vi "Shutter Experiments.vi"(8 "Laser Shutter":enum32{"GFP", "Cy3 Long Pass", "Cy3", "Cy5"}(radio)) -> ()   [LabVIEW 2014]
uses:
  global current shutter.vi
panel:
  out "Current Wheel Position":string
  in  "Wheel Speed":u8=1 min=1 max=7 step=1
  in  "stop":bool
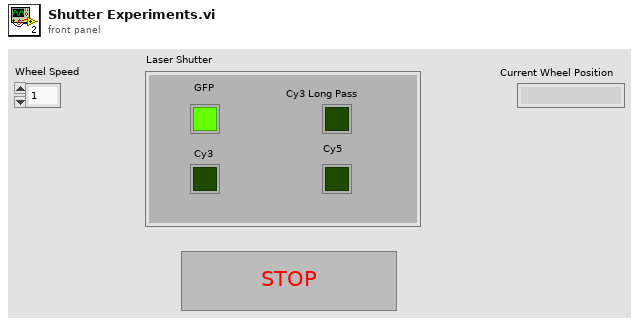
[diagram p1: front panel]
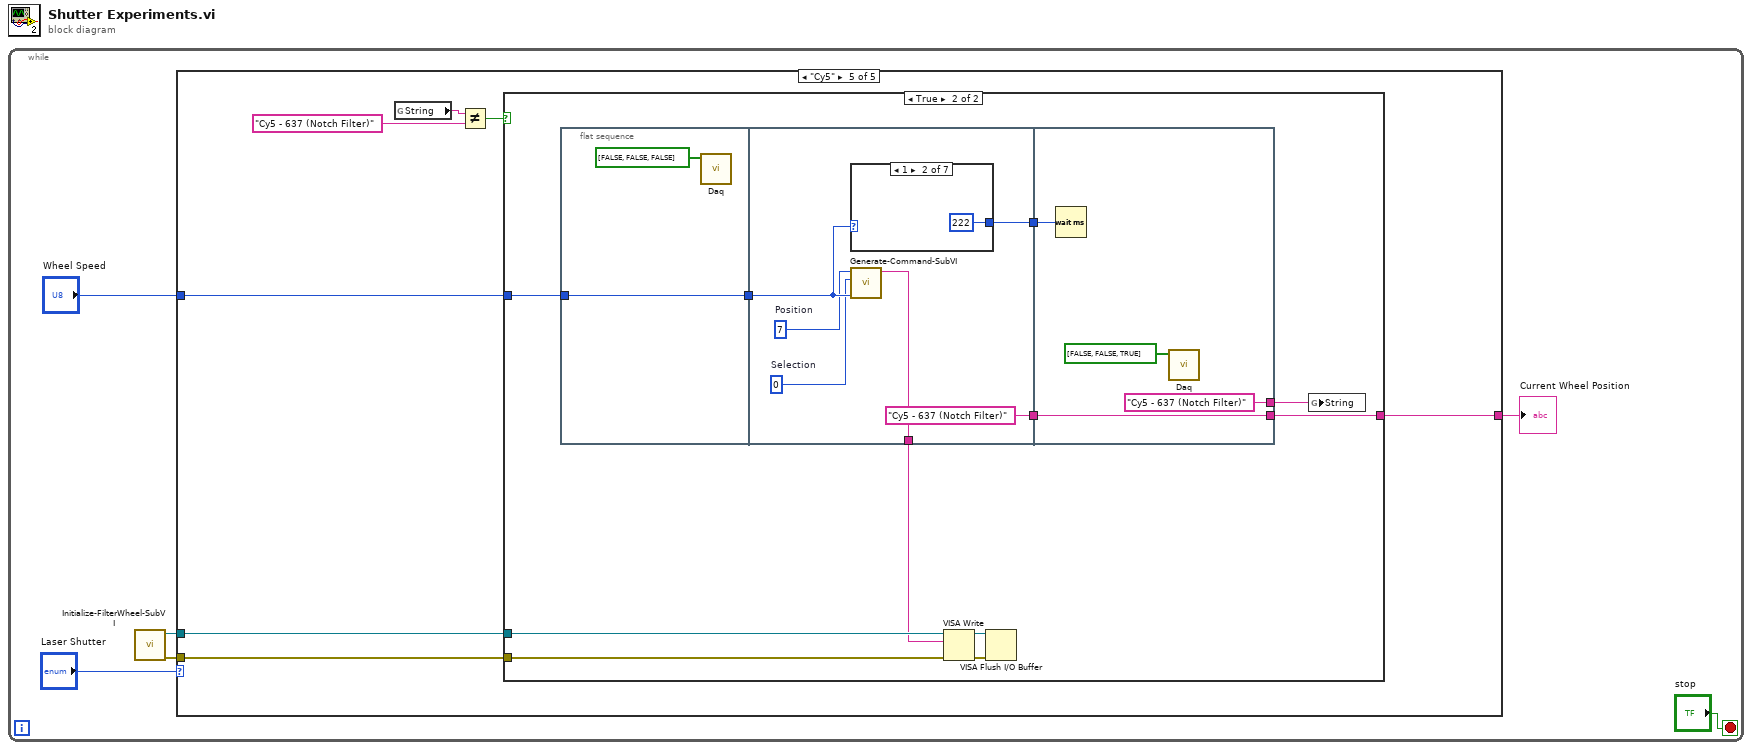
[diagram p0: block diagram]
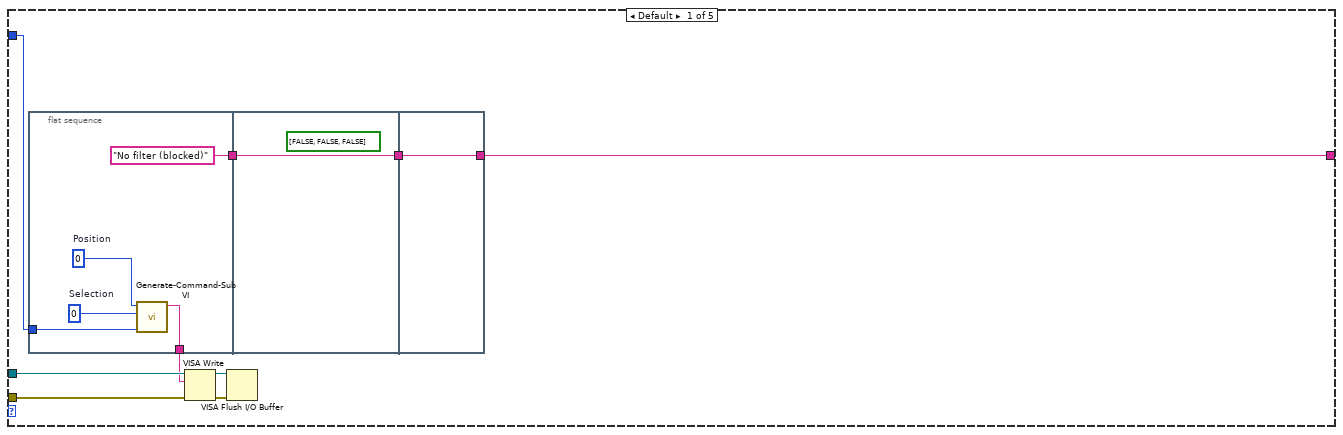
[diagram p2: hidden frame]
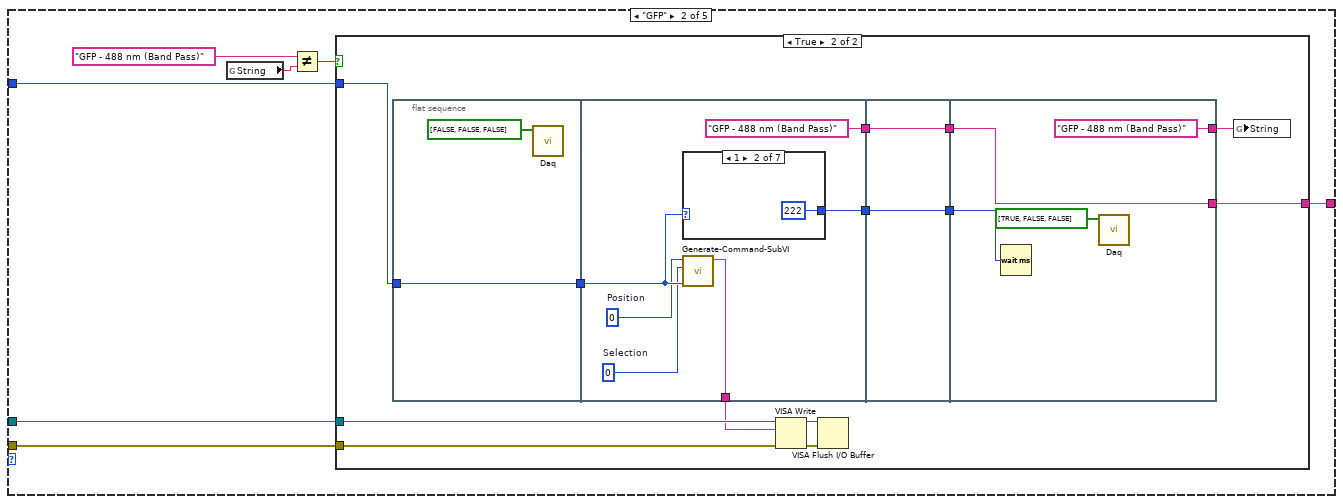
[diagram p3: hidden frame]
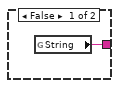
[diagram p4: hidden frame]
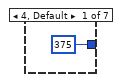
[diagram p5: hidden frame]
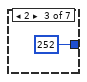
[diagram p6: hidden frame]
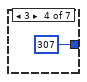
[diagram p7: hidden frame]
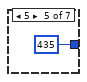
[diagram p8: hidden frame]
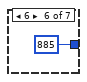
[diagram p9: hidden frame]
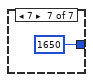
[diagram p10: hidden frame]
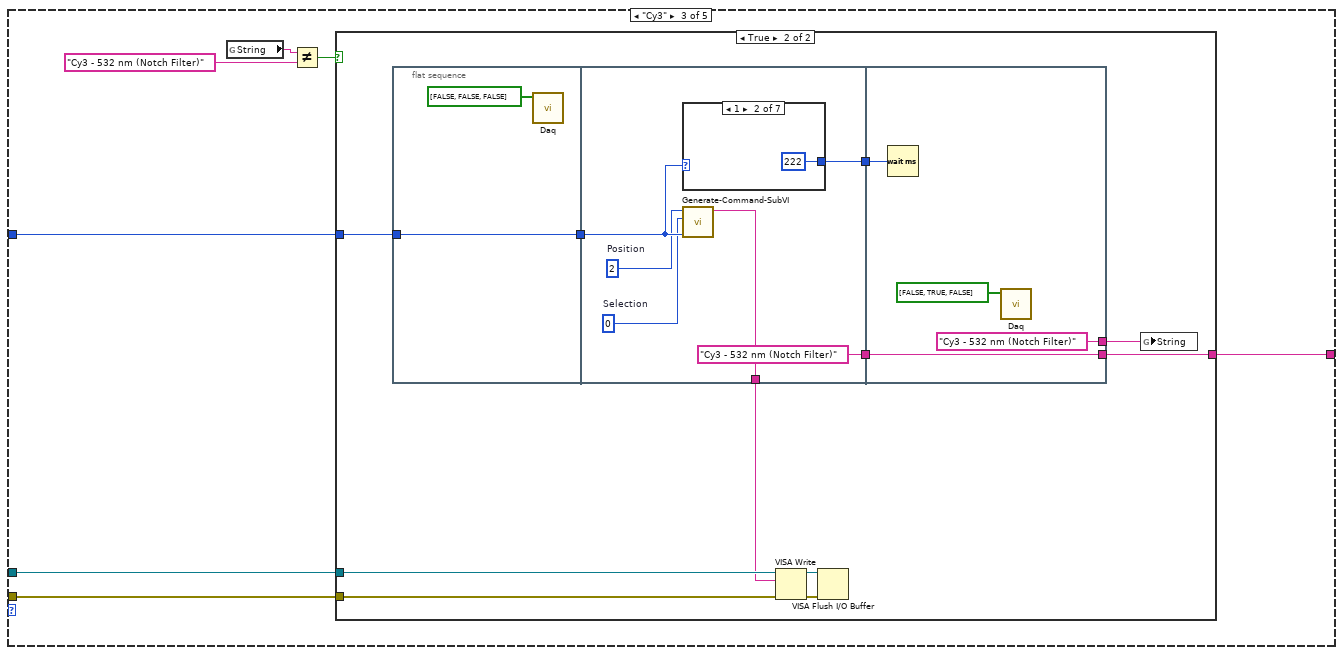
[diagram p11: hidden frame]
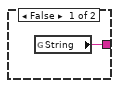
[diagram p12: hidden frame]
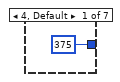
[diagram p13: hidden frame]
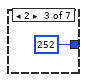
[diagram p14: hidden frame]
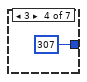
[diagram p15: hidden frame]
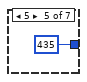
[diagram p16: hidden frame]
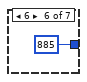
[diagram p17: hidden frame]
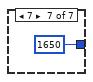
[diagram p18: hidden frame]
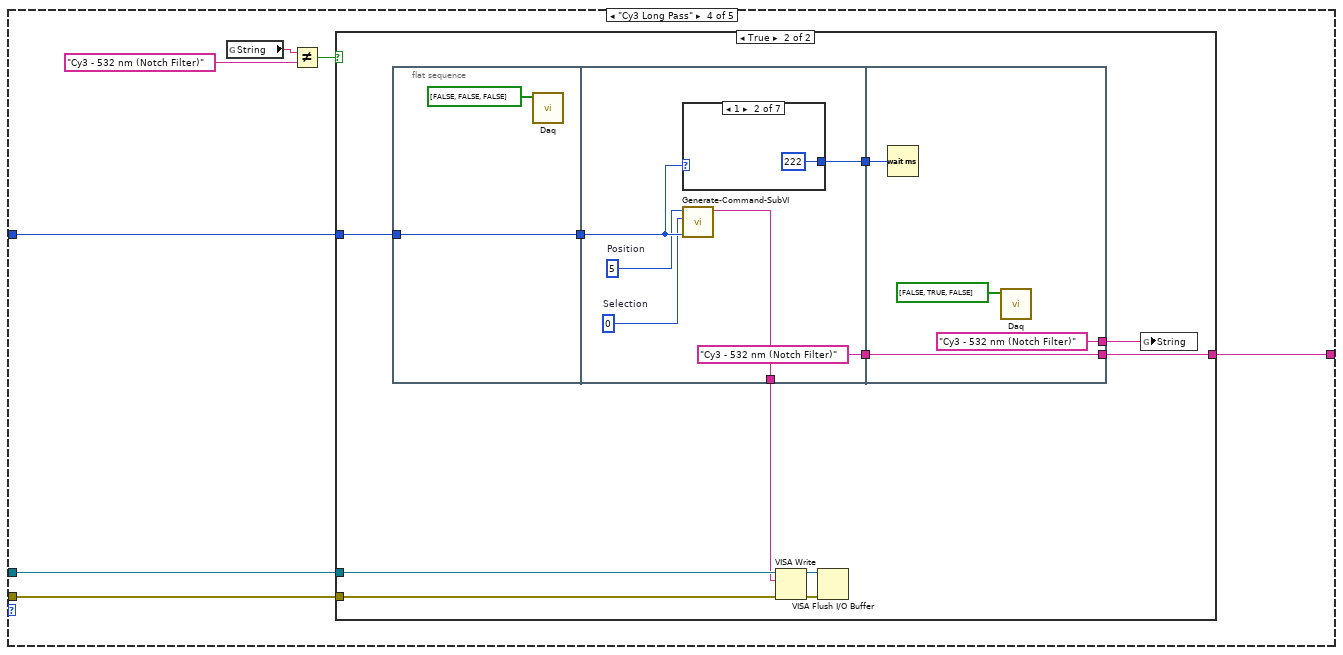
[diagram p19: hidden frame]
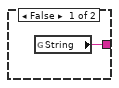
[diagram p20: hidden frame]
diagram:
  n1 = while {
    stop <- "stop" stop-if-true
    n2 = call <userlib>:"Initialize-FilterWheel-SubVI.vi"() -> ("VISA resource name out"=w3:refnum<visa-resource-name>, "error out"=w2:errorcluster)  [unwired: 9 in]
    n3 = case shown="\"Cy5\"" "Laser Shutter" {
      tunnel: "Wheel Speed" -> [w15 w29 w71 w109 w147]
      tunnel: w3 -> [w12 w28 w70 w108 w146]
      tunnel: w2 -> [w11 w27 w69 w107 w145]
      tunnel: [w9 w26 w68 w106 w144] -> w1
      frame Default {
        n4 = flat-sequence {
          tunnel: w15 -> [w20]
          tunnel: [w17] -> w10
          tunnel: ["No filter (blocked)"] -> w8
          tunnel: w8 -> [w21]
          tunnel: [w21] -> w7
          tunnel: [w22] -> w9
          tunnel: w7 -> [w22]
          frame #0 {
            w18 = 0  # Selection
            w19 = 0  # Position
            n5 = call <userlib>:"Generate-Command-SubVI.vi"("Wheel Speed"=w20, "Wheel Selection"=w18, "Wheel Position"=w19) -> ("type"=w17:string)  [unwired: 8 in]
          }
          frame #1 {
            (unwired) bool[] [FALSE, FALSE, FALSE]
          }
          frame #2 {
          }
        }
        n6 = VISA Write(VISA resource name=w12, write buffer=w10, error in (no error)=w11) -> (VISA resource name out=w13:refnum<visa-resource-name>, error out=w14:errorcluster)  [unwired: 1 out]
        n7 = VISA Flush I/O Buffer(VISA resource name=w13, error in (no error)=w14) -> ()  [unwired: 1 in, 2 out]
      }
      frame "GFP" {
        n8 = global read "global current shutter.vi" "String"() -> (w24:string)
        n9 = Not Equal?(x="GFP - 488 nm (Band Pass)", y=w24) -> (x != y?=w23:bool)
        n10 = case shown="True" w23 {
          tunnel: w29 -> [_ w38]
          tunnel: w28 -> [_ w35]
          tunnel: w27 -> [_ w34]
          tunnel: [w30 w32] -> w26
          frame False {
            n11 = global read "global current shutter.vi" "String"() -> (w30:string)
          }
          frame True {
            n12 = flat-sequence {
              tunnel: w38 -> [w45]
              tunnel: [w45] -> w43
              tunnel: [w48] -> w42
              tunnel: [w47] -> w33
              tunnel: ["GFP - 488 nm (Band Pass)"] -> w41
              tunnel: w43 -> [w51]
              tunnel: w42 -> [w59]
              tunnel: w41 -> [w60]
              tunnel: [w60] -> w40
              tunnel: [w59] -> w39
              tunnel: [w62] -> w32
              tunnel: w40 -> [w62]
              tunnel: w39 -> [w64]
              tunnel: ["GFP - 488 nm (Band Pass)"] -> w31
              frame #0 {
                n13 = call "Daq.vi"("Array"=bool[] [FALSE, FALSE, FALSE]) -> ()  [unwired: 11 in]
              }
              frame #1 {
                w49 = 0  # Selection
                w50 = 0  # Position
                n14 = case shown="1" w51 {
                  tunnel: [375 222 252 307 435 885 1650] -> w48
                  frame 4, Default {
                  }
                  frame 1 {
                  }
                  frame 2 {
                  }
                  frame 3 {
                  }
                  frame 5 {
                  }
                  frame 6 {
                  }
                  frame 7 {
                  }
                }
                n15 = call <userlib>:"Generate-Command-SubVI.vi"("Wheel Speed"=w51, "Wheel Selection"=w49, "Wheel Position"=w50) -> ("type"=w47:string)  [unwired: 8 in]
              }
              frame #2 {
              }
              frame #3 {
                n16 = Wait (ms)(milliseconds to wait=w64) -> ()  [unwired: 1 out]
                n17 = call "Daq.vi"("Array"=bool[] [TRUE, FALSE, FALSE]) -> ()  [unwired: 11 in]
              }
            }
            n18 = VISA Write(VISA resource name=w35, write buffer=w33, error in (no error)=w34) -> (VISA resource name out=w37:refnum<visa-resource-name>, error out=w36:errorcluster)  [unwired: 1 out]
            n19 = VISA Flush I/O Buffer(VISA resource name=w37, error in (no error)=w36) -> ()  [unwired: 1 in, 2 out]
            n20 = global write "global current shutter.vi" "String"(w31) -> ()
          }
        }
      }
      frame "Cy3" {
        n21 = global read "global current shutter.vi" "String"() -> (w66:string)
        n22 = Not Equal?(x=w66, y="Cy3 - 532 nm (Notch Filter)") -> (x != y?=w65:bool)
        n23 = case shown="True" w65 {
          tunnel: w71 -> [_ w80]
          tunnel: w70 -> [_ w77]
          tunnel: w69 -> [_ w76]
          tunnel: [w72 w74] -> w68
          frame False {
            n24 = global read "global current shutter.vi" "String"() -> (w72:string)
          }
          frame True {
            n25 = flat-sequence {
              tunnel: w80 -> [w85]
              tunnel: [w85] -> w83
              tunnel: [w88] -> w82
              tunnel: [w87] -> w75
              tunnel: ["Cy3 - 532 nm (Notch Filter)"] -> w81
              tunnel: w83 -> [w91]
              tunnel: w82 -> [w102]
              tunnel: [w101] -> w74
              tunnel: w81 -> [w101]
              tunnel: ["Cy3 - 532 nm (Notch Filter)"] -> w73
              frame #0 {
                n26 = call "Daq.vi"("Array"=bool[] [FALSE, FALSE, FALSE]) -> ()  [unwired: 11 in]
              }
              frame #1 {
                w89 = 0  # Selection
                w90 = 2  # Position
                n27 = case shown="1" w91 {
                  tunnel: [375 222 252 307 435 885 1650] -> w88
                  frame 4, Default {
                  }
                  frame 1 {
                  }
                  frame 2 {
                  }
                  frame 3 {
                  }
                  frame 5 {
                  }
                  frame 6 {
                  }
                  frame 7 {
                  }
                }
                n28 = call <userlib>:"Generate-Command-SubVI.vi"("Wheel Speed"=w91, "Wheel Selection"=w89, "Wheel Position"=w90) -> ("type"=w87:string)  [unwired: 8 in]
              }
              frame #2 {
                n29 = Wait (ms)(milliseconds to wait=w102) -> ()  [unwired: 1 out]
                n30 = call "Daq.vi"("Array"=bool[] [FALSE, TRUE, FALSE]) -> ()  [unwired: 11 in]
              }
            }
            n31 = VISA Write(VISA resource name=w77, write buffer=w75, error in (no error)=w76) -> (VISA resource name out=w79:refnum<visa-resource-name>, error out=w78:errorcluster)  [unwired: 1 out]
            n32 = VISA Flush I/O Buffer(VISA resource name=w79, error in (no error)=w78) -> ()  [unwired: 1 in, 2 out]
            n33 = global write "global current shutter.vi" "String"(w73) -> ()
          }
        }
      }
      frame "Cy3 Long Pass" {
        n34 = global read "global current shutter.vi" "String"() -> (w105:string)
        n35 = Not Equal?(x=w105, y="Cy3 - 532 nm (Notch Filter)") -> (x != y?=w103:bool)
        n36 = case shown="True" w103 {
          tunnel: w109 -> [_ w118]
          tunnel: w108 -> [_ w115]
          tunnel: w107 -> [_ w114]
          tunnel: [w110 w112] -> w106
          frame False {
            n37 = global read "global current shutter.vi" "String"() -> (w110:string)
          }
          frame True {
            n38 = flat-sequence {
              tunnel: w118 -> [w123]
              tunnel: [w123] -> w121
              tunnel: [w126] -> w120
              tunnel: [w125] -> w113
              tunnel: ["Cy3 - 532 nm (Notch Filter)"] -> w119
              tunnel: w121 -> [w129]
              tunnel: w120 -> [w140]
              tunnel: [w139] -> w112
              tunnel: w119 -> [w139]
              tunnel: ["Cy3 - 532 nm (Notch Filter)"] -> w111
              frame #0 {
                n39 = call "Daq.vi"("Array"=bool[] [FALSE, FALSE, FALSE]) -> ()  [unwired: 11 in]
              }
              frame #1 {
                w127 = 0  # Selection
                w128 = 5  # Position
                n40 = case shown="1" w129 {
                  tunnel: [375 222 252 307 435 885 1650] -> w126
                  frame 4, Default {
                  }
                  frame 1 {
                  }
                  frame 2 {
                  }
                  frame 3 {
                  }
                  frame 5 {
                  }
                  frame 6 {
                  }
                  frame 7 {
                  }
                }
                n41 = call <userlib>:"Generate-Command-SubVI.vi"("Wheel Speed"=w129, "Wheel Selection"=w127, "Wheel Position"=w128) -> ("type"=w125:string)  [unwired: 8 in]
              }
              frame #2 {
                n42 = Wait (ms)(milliseconds to wait=w140) -> ()  [unwired: 1 out]
                n43 = call "Daq.vi"("Array"=bool[] [FALSE, TRUE, FALSE]) -> ()  [unwired: 11 in]
              }
            }
            n44 = VISA Write(VISA resource name=w115, write buffer=w113, error in (no error)=w114) -> (VISA resource name out=w117:refnum<visa-resource-name>, error out=w116:errorcluster)  [unwired: 1 out]
            n45 = VISA Flush I/O Buffer(VISA resource name=w117, error in (no error)=w116) -> ()  [unwired: 1 in, 2 out]
            n46 = global write "global current shutter.vi" "String"(w111) -> ()
          }
        }
      }
      frame "Cy5" {
        n47 = global read "global current shutter.vi" "String"() -> (w143:string)
        n48 = Not Equal?(x=w143, y="Cy5 - 637 (Notch Filter)") -> (x != y?=w141:bool)
        n49 = case shown="True" w141 {
          tunnel: w147 -> [_ w156]
          tunnel: w146 -> [_ w153]
          tunnel: w145 -> [_ w152]
          tunnel: [w148 w150] -> w144
          frame False {
            n50 = global read "global current shutter.vi" "String"() -> (w148:string)
          }
          frame True {
            n51 = flat-sequence {
              tunnel: w156 -> [w161]
              tunnel: [w161] -> w159
              tunnel: [w164] -> w158
              tunnel: [w163] -> w151
              tunnel: ["Cy5 - 637 (Notch Filter)"] -> w157
              tunnel: w159 -> [w167]
              tunnel: w158 -> [w178]
              tunnel: [w177] -> w150
              tunnel: w157 -> [w177]
              tunnel: ["Cy5 - 637 (Notch Filter)"] -> w149
              frame #0 {
                n52 = call "Daq.vi"("Array"=bool[] [FALSE, FALSE, FALSE]) -> ()  [unwired: 11 in]
              }
              frame #1 {
                w165 = 0  # Selection
                w166 = 7  # Position
                n53 = case shown="1" w167 {
                  tunnel: [375 222 252 307 435 885 1650] -> w164
                  frame 4, Default {
                  }
                  frame 1 {
                  }
                  frame 2 {
                  }
                  frame 3 {
                  }
                  frame 5 {
                  }
                  frame 6 {
                  }
                  frame 7 {
                  }
                }
                n54 = call <userlib>:"Generate-Command-SubVI.vi"("Wheel Speed"=w167, "Wheel Selection"=w165, "Wheel Position"=w166) -> ("type"=w163:string)  [unwired: 8 in]
              }
              frame #2 {
                n55 = Wait (ms)(milliseconds to wait=w178) -> ()  [unwired: 1 out]
                n56 = call "Daq.vi"("Array"=bool[] [FALSE, FALSE, TRUE]) -> ()  [unwired: 11 in]
              }
            }
            n57 = VISA Write(VISA resource name=w153, write buffer=w151, error in (no error)=w152) -> (VISA resource name out=w155:refnum<visa-resource-name>, error out=w154:errorcluster)  [unwired: 1 out]
            n58 = VISA Flush I/O Buffer(VISA resource name=w155, error in (no error)=w154) -> ()  [unwired: 1 in, 2 out]
            n59 = global write "global current shutter.vi" "String"(w149) -> ()
          }
        }
      }
    }
    "Current Wheel Position" <- w1
  }
